vi "current-instance.vi"() -> ()   [LabVIEW 2016, in "test-Application.lvlib"]
uses:
  test-Application.lvlib
  <vilib>/addons/_JKI Toolkits/Caraya/classes/Assert/Assert Equal Value_Variant.vi
  <vilib>/addons/_JKI Toolkits/Caraya/classes/Test/Test.lvclass
  <vilib>/addons/_JKI Toolkits/Caraya/classes/Assert/Assert.lvclass
  main/apis/Application/Application.lvclass
panel:
  out "error out":errorcluster
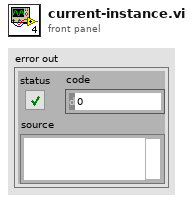
[diagram p1: front panel]
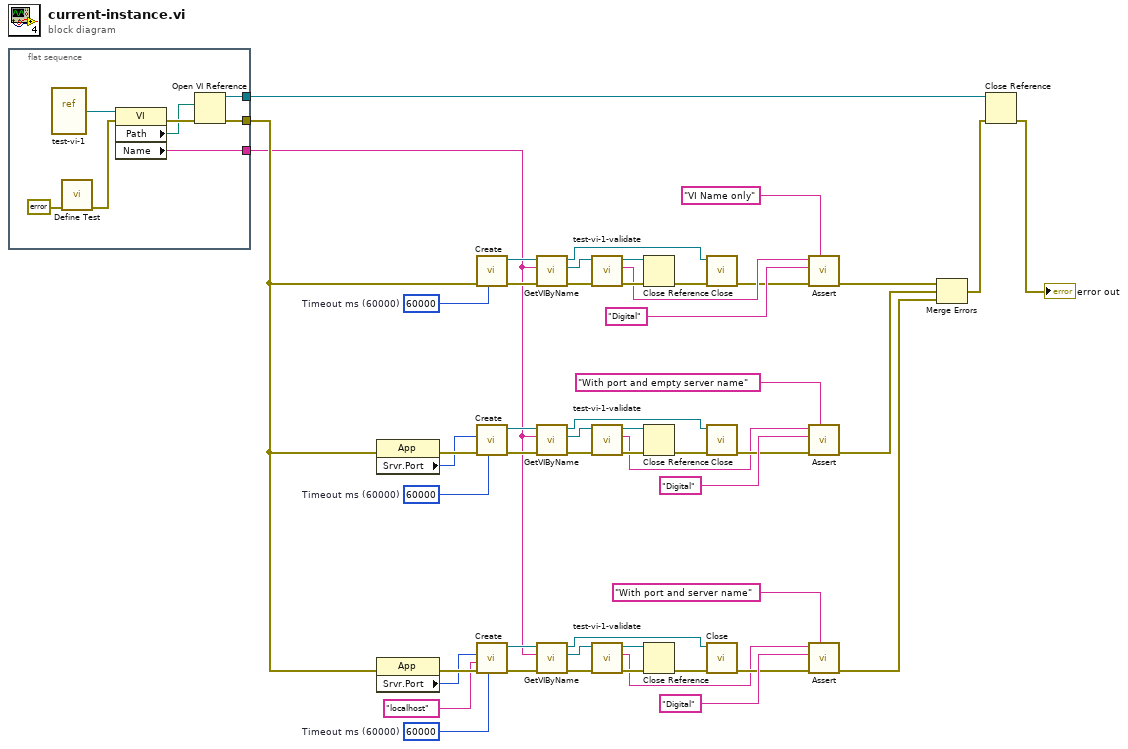
[diagram p0: block diagram]
diagram:
  w3 = 60000  # Timeout ms (60000)
  w16 = 60000  # Timeout ms (60000)
  w38 = 60000  # Timeout ms (60000)
  n1 = flat-sequence {
    tunnel: [w56] -> w33
    tunnel: [w55] -> w39
    tunnel: [w53] -> w1
    frame #0 {
      n2 = vi-ref "test-vi-1.vi"() -> (w58:refnum<vi>)
      n3 = call <vilib>:"Define Test.vi"("error in (no error)"=errorcluster {"status"=FALSE, "code"=0, "source"=""}) -> ("error out"=w59:errorcluster)  [unwired: 10 in]
      n4 = property on="Property Node" class="VI"(reference=w58, error in=w59) -> (error out=w57:errorcluster, "Path"=w54:path, "Name"=w53:string)  [unwired: 1 out]
      n5 = Open VI Reference(vi path=w54, error in (no error)=w57) -> (vi reference=w55:refnum<vi>, error out=w56:errorcluster)  [unwired: 4 in]
    }
  }
  n6 = property on="Property Node" class="App"(error in=w33) -> (error out=w20:errorcluster, "Srvr.Port"=w17:u32)  [unwired: 1 in, 1 out]
  n7 = property on="Property Node" class="App"(error in=w33) -> (error out=w7:errorcluster, "Srvr.Port"=w5:u32)  [unwired: 1 in, 1 out]
  n8 = call "Create.vi"("Timeout ms (60000)"=w38, "error in (no error)"=w33) -> ("error out"=w32:errorcluster, "Application out"=w36:refnum<class "Application.lvclass">)  [unwired: 8 in]
  n9 = call "Create.vi"("Timeout ms (60000)"=w16, "error in (no error)"=w20, "Port(0:Ignored)"=w17) -> ("error out"=w27:errorcluster, "Application out"=w24:refnum<class "Application.lvclass">)  [unwired: 7 in]
  n10 = call "Create.vi"("Timeout ms (60000)"=w3, "error in (no error)"=w7, "Service Name (\"\":localhost)"="localhost" ("Service Name (\"\":localhost)"), "Port(0:Ignored)"=w5) -> ("error out"=w9:errorcluster, "Application out"=w12:refnum<class "Application.lvclass">)  [unwired: 6 in]
  n11 = call "GetVIByName.vi"("error in (no error)"=w32, "VI Name"=w1, "Application in"=w36) -> ("error out"=w37:errorcluster, "VI Reference"=w34:refnum<vi>, "Application out"=w35:refnum<class "Application.lvclass">)  [unwired: 6 in]
  n12 = call "GetVIByName.vi"("error in (no error)"=w27, "VI Name"=w1, "Application in"=w24) -> ("error out"=w23:errorcluster, "VI Reference"=w26:refnum<vi>, "Application out"=w25:refnum<class "Application.lvclass">)  [unwired: 6 in]
  n13 = call "GetVIByName.vi"("error in (no error)"=w9, "VI Name"=w1, "Application in"=w12) -> ("error out"=w13:errorcluster, "VI Reference"=w10:refnum<vi>, "Application out"=w11:refnum<class "Application.lvclass">)  [unwired: 6 in]
  n14 = call "test-vi-1-validate.vi"("error in (no error)"=w37, "VI in"=w34) -> ("error out"=w50:errorcluster, "ClassName"=w48:string, "VI out"=w49:refnum<vi>)  [unwired: 7 in]
  n15 = call "test-vi-1-validate.vi"("error in (no error)"=w23, "VI in"=w26) -> ("error out"=w21:errorcluster, "ClassName"=w18:string, "VI out"=w22:refnum<vi>)  [unwired: 7 in]
  n16 = call "test-vi-1-validate.vi"("error in (no error)"=w13, "VI in"=w10) -> ("error out"=w15:errorcluster, "ClassName"=w2:string, "VI out"=w14:refnum<vi>)  [unwired: 7 in]
  n17 = Close Reference(reference=w49, error in (no error)=w50) -> (error out=w30:errorcluster)
  n18 = Close Reference(reference=w22, error in (no error)=w21) -> (error out=w28:errorcluster)
  n19 = Close Reference(reference=w14, error in (no error)=w15) -> (error out=w8:errorcluster)
  n20 = call "Close.vi"("error in (no error)"=w30, "Application in"=w35) -> ("error out"=w29:errorcluster)  [unwired: 9 in]
  n21 = call "Close.vi"("error in (no error)"=w28, "Application in"=w25) -> ("error out"=w19:errorcluster)  [unwired: 9 in]
  n22 = call "Close.vi"("error in (no error)"=w8, "Application in"=w11) -> ("error out"=w6:errorcluster)  [unwired: 9 in]
  n23 = call-poly <vilib>:"Assert.vi"("Label"="VI Name only" ("Label (VI Title)"), "error in (no error)"=w29, "Y"="Digital" ("Class Name"), "X"=w48) -> ("error out"=w51:errorcluster)  [unwired: 7 in]
  n24 = call-poly <vilib>:"Assert.vi"("Label"="With port and empty server name" ("Label (VI Title)"), "error in (no error)"=w19, "Y"="Digital" ("Class Name"), "X"=w18) -> ("error out"=w44:errorcluster)  [unwired: 7 in]
  n25 = call-poly <vilib>:"Assert.vi"("Label"="With port and server name" ("Label (VI Title)"), "error in (no error)"=w6, "Y"="Digital" ("Class Name"), "X"=w2) -> ("error out"=w41:errorcluster)  [unwired: 7 in]
  n26 = Merge Errors(w51, w44, w41) -> (w31:errorcluster)
  n27 = Close Reference(reference=w39, error in (no error)=w31) -> (error out=→"error out":errorcluster)
